vi "Assert Session Exists.vi"(8 "error in":errorcluster, 10 "expected value":bool=TRUE, 11 "session reservation in":refnum<class "Session Reservation.lvclass">) -> (0 "error out":errorcluster, 1 "result":string, 2 "pass":bool, 3 "session reservation out":refnum<class "Session Reservation.lvclass">)   [LabVIEW 2020, in "MeasurementServerTests.lvlib" / "Session Reservation Tests.lvlib"]
uses:
  Session Reservation Tests.lvlib
  Runtime/MeasurementLink Session Management/Session Reservation/Session Reservation.lvclass
  Runtime/MeasurementLink Session Management/Session Reservation/Session Reservation.lvclass/Session Reservation.ctl
  Runtime/MeasurementLink Session Management/Session Reservation/Get Session Info - NSess .vi
  Runtime/MeasurementLink Session Management/Session Reservation/Merge Invalid DVR Error.vi
  Runtime/MeasurementLink Session Management/Session Reservation/Is DVR Valid.vi
  Runtime/MeasurementLink Measurement Server/Helpers/Error Strings Global Internal.vi
  <vilib>/Utility/error.llb/Error Cluster From Error Code.vi
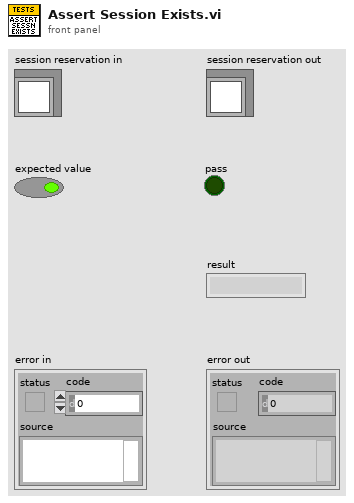
[diagram p1: front panel]
types:
  T1 = typedef "MeasurementLink Session Management Client.lvlib/ni_measurementlink_sessionmanagement_v1_SessionInformation.ctl" = cluster{"session":T2, "resource_name":string, "channel_list":string, "instrument_type_id":string, "session_exists":bool, "channel_mappings":T3[]}
  T2 = typedef "MeasurementLink Session Management Client.lvlib/nidevice_grpc_Session.ctl" = cluster{"name":string}
  T3 = typedef "MeasurementLink Session Management Client.lvlib/ni_measurementlink_sessionmanagement_v1_ChannelMapping.ctl" = cluster{"pin_or_relay_name":string, "site":i32, "channel":string}
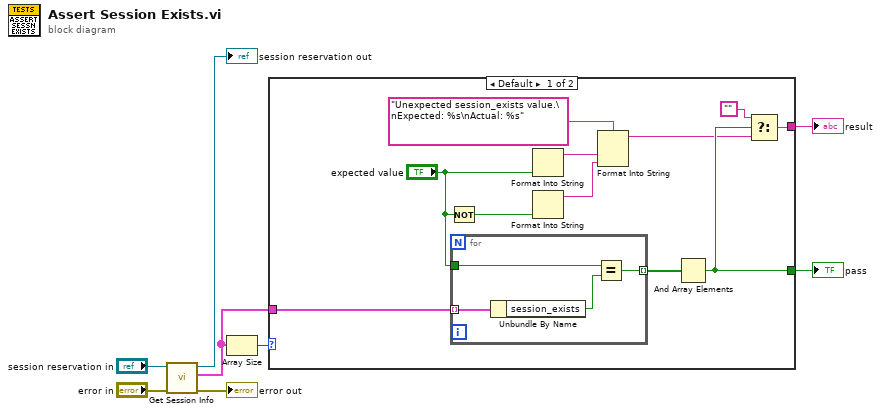
[diagram p0: block diagram]
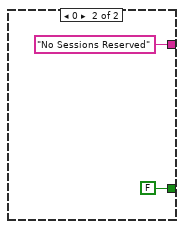
[diagram p2: hidden frame]
diagram:
  n1 = call-poly "Get Session Info.vi"("error in"="error in", "session reservation in"="session reservation in") -> ("error out"=→"error out":errorcluster, "sessions info"=w1:T1[], "session reservation out"=→"session reservation out":refnum<class "Session Reservation.lvclass">)  [unwired: 7 in]
  n2 = Array Size(array=w1) -> (size(s)=w4:i32)
  n3 = case shown="Default" w4 {
    tunnel: [w17 FALSE ("pass")] -> w3
    tunnel: [w16 "No Sessions Reserved"] -> w2
    tunnel: w1 -> [w18 _]
    frame Default {
      n4 = Not(x="expected value") -> (.not. x?=w11:bool)
      n5 = for {
        tunnel: w18 -> [w23] mode=indexing
        tunnel: [w21] -> w19 mode=indexing
        tunnel: "expected value" -> [w20]
        n6 = Unbundle By Name(w23) -> ("session_exists"=w22:bool)
        n7 = Equal?(x=w20, y=w22) -> (x = y?=w21:bool)
      }
      n8 = Format Into String("expected value") -> (resulting string=w13:string)  [unwired: 3 in, 1 out]
      n9 = Format Into String(w11) -> (resulting string=w12:string)  [unwired: 3 in, 1 out]
      n10 = Format Into String(format string="Unexpected session_exists value.\nExpected: %s\nActual: %s", w13, w12) -> (resulting string=w9:string)  [unwired: 2 in, 1 out]
      n11 = And Array Elements(Boolean array=w19) -> (logical AND=w17:bool)
      n12 = Select(t="", s=w17, f=w9) -> (s? t:f=w16:string)
    }
    frame 0 {
    }
  }
  "pass" <- w3
  "result" <- w2
